vi "ST Hear.vi"(5 "VISA resource name":refnum<visa-resource-name>, 6 "Time Out":i32, 7 "error in (no error)":errorcluster) -> (0 "VISA resource name out":refnum<visa-resource-name>, 1 "String Received":string, 2 "Result Code":i32, 3 "error out":errorcluster, 4 "Ready and OK":bool)   [LabVIEW 2009]
doc: "The VI reads the return string from a ST Send operation. The result out has the following meaning:\n 0 >>> Operation not complete\n 1 >>> Operation Complete with an Error\n 2 >>> Operation Complete without Error\n-1 >>> Operation caused a Communication Error"
panel:
  out "Ready with Error":bool
  out "Time Out":bool
  out "Com Error":bool
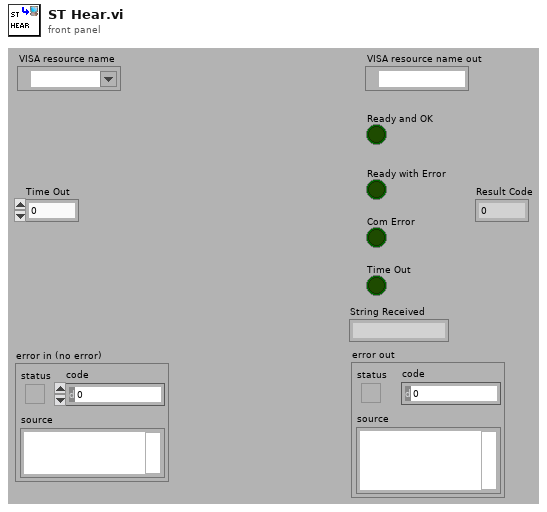
[diagram p1: front panel]
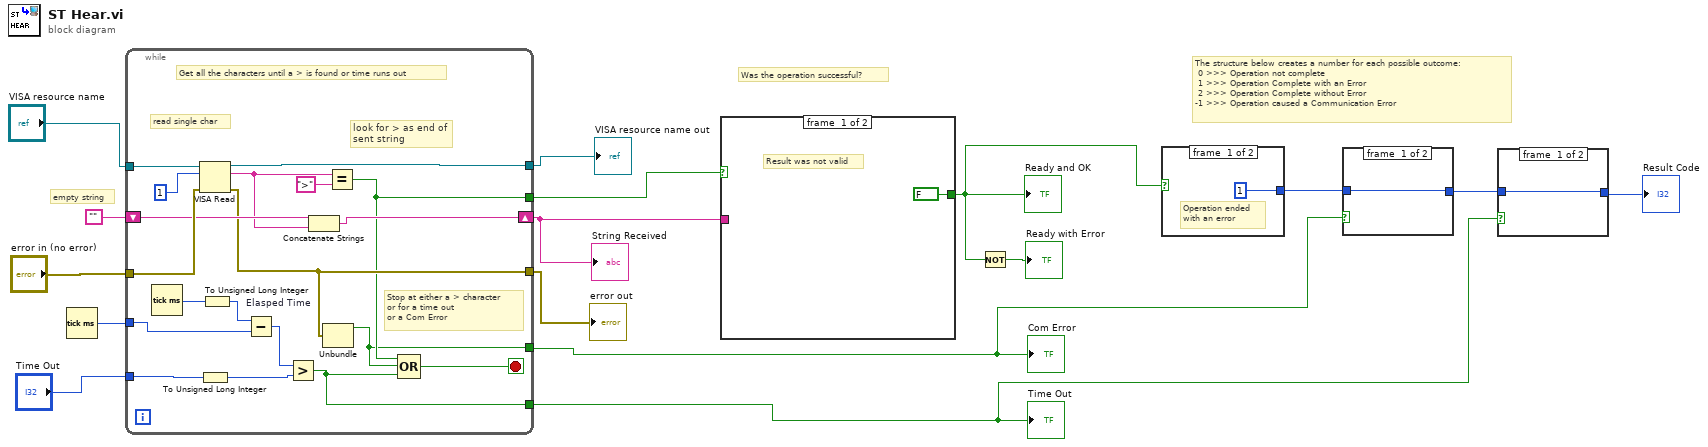
[diagram p0: block diagram]
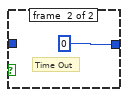
[diagram p2: hidden frame]
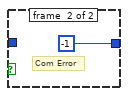
[diagram p3: hidden frame]
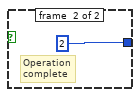
[diagram p4: hidden frame]
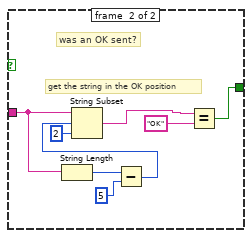
[diagram p5: hidden frame]
diagram:
  # "The structure below creates a number for each possible outcome:\n 0 >>> Operation not complete\n 1 >>> Operation Complete with an Error\n 2 >>> Operation Complete without Error\n-1 >>> Operation caused a Communication Error"
  # "Was the operation successful?"
  # "empty string"
  n1 = Tick Count (ms)() -> (millisecond timer value=w12:u32)
  n2 = while {
    tunnel: "VISA resource name" -> [w35]
    tunnel: "error in (no error)" -> [w34]
    tunnel: [w21] -> w8
    tunnel: [w32] -> w14
    shift-right: [w28] -> w9
    shift-left: "" -> [w30]
    tunnel: w12 -> [w27]
    tunnel: "Time Out" -> [w26]
    tunnel: [w18] -> w10
    tunnel: [w20] -> w3
    tunnel: [w17] -> w4
    stop <- w19 stop-if-true
    # "Get all the characters until a > is found or time runs out"
    # "Stop at either a > character\nor for a time out \nor a Com Error"
    # "look for > as end of \nsent string"
    # "read single char"
    n3 = Tick Count (ms)() -> (millisecond timer value=w24:u32)
    n4 = VISA Read(VISA resource name=w35, byte count=u32 1, error in (no error)=w34) -> (VISA resource name out=w32:refnum<visa-resource-name>, read buffer=w29:string, error out=w21:errorcluster)  [unwired: 1 out]
    n5 = To Unsigned Long Integer(number=w26) -> (unsigned 32bit integer=w25:u32)
    n6 = To Unsigned Long Integer(number=w24) -> (unsigned 32bit integer=w23:u32)
    n7 = Subtract "Elasped Time"(x=w23, y=w27) -> (x-y=w22:u32)
    n8 = Greater?(x=w22, y=w25) -> (0:w20:bool)
    n9 = Concatenate Strings(w30, w29) -> (w28:string)
    n10 = Unbundle(w21) -> ("status"=w17:bool)  [unwired: 2 out]
    n11 = Equal?(x=w29, y=">") -> (x = y?=w18:bool)
    n12 = Compound Arithmetic op=OR(w18, w17, w20) -> (w19:bool)
  }
  "error out" <- w8
  "VISA resource name out" <- w14
  "String Received" <- w9
  "Com Error" <- w4
  "Time Out" <- w3
  n13 = case shown="True" w10 {
    tunnel: w9 -> [_ w44]
    tunnel: [FALSE w37] -> w7
    frame #0 {
      # "Result was not valid"
    }
    frame #1 {
      # "get the string in the OK position"
      # "was an OK sent?"
      n14 = String Length(string=w44) -> (length=w43:i32)
      n15 = Subtract(x=w43, y=5) -> (x-y=w41:i32)
      n16 = String Subset(string=w44, offset (0)=w41, length (rest)=2 ("length (rest)")) -> (substring=w38:string)
      n17 = Equal?(x=w38, y="OK" ("regular expression")) -> (x = y?=w37:bool)
    }
  }
  "Ready and OK" <- w7
  n18 = Not(x=w7) -> (.not. x?=→"Ready with Error":bool)
  n19 = case shown="True" w7 {
    tunnel: [1 2] -> w5
    frame #0 {
      # "Operation ended\nwith an error"
    }
    frame #1 {
      # "Operation \ncomplete"
    }
  }
  n20 = case shown="True" w4 {
    tunnel: w5 -> [w47 _]
    tunnel: [w47 -1] -> w2
    frame #0 {
    }
    frame #1 {
      # "Com Error"
    }
  }
  n21 = case shown="True" w3 {
    tunnel: w2 -> [w49 _]
    tunnel: [w49 0] -> w1
    frame #0 {
    }
    frame #1 {
      # "Time Out"
    }
  }
  "Result Code" <- w1
